vi "CM_Packet_To_Processed_Bytes.vi"(3 "error in (no error)":errorcluster, 4 "CM Params":T5, 5 "CM Packet In":T1) -> (0 "error out":errorcluster, 1 "Processed Bytes":u8[](array[numeric]), 2 "CM Packet Out":T1)   [LabVIEW 2017]
uses:
  Controls/Packet/Packet.ctl
  Controls/Packet/Packet_Direction.ctl
  Controls/Packet/Packet_Type.ctl
  Controls/Packet/Packet_Priority.ctl
  Controls/Control Packets/CM_Param.ctl
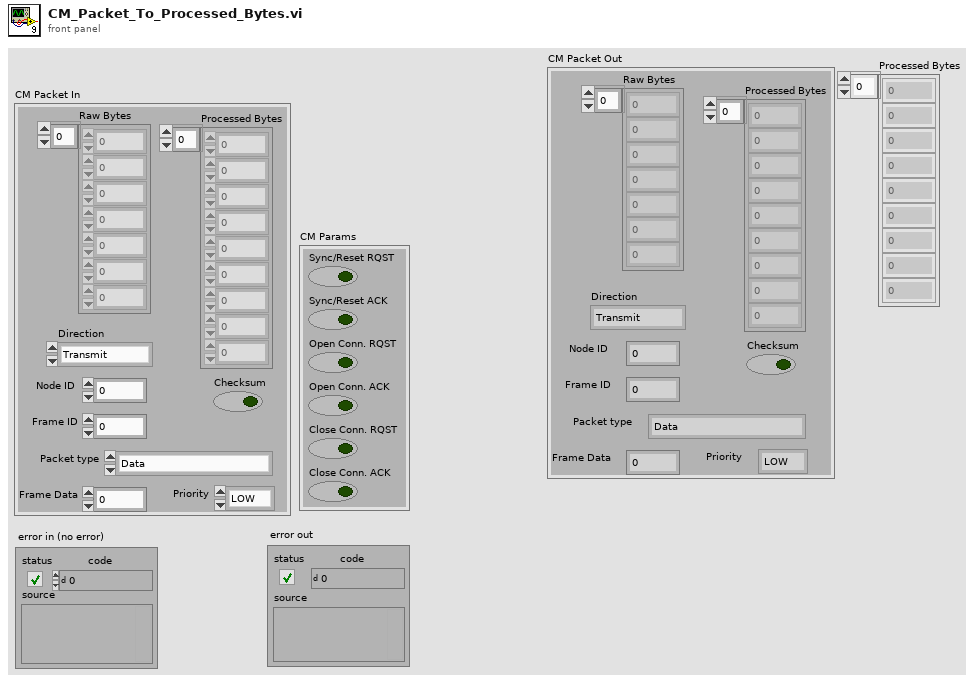
[diagram p1: front panel]
types:
  T1 = typedef "Packet.ctl" = cluster{"Raw Bytes":u8[], "Checksum":bool, "Direction":T2, "Processed Bytes":u8[], "Node ID":u8, "Packet type":T3, "Frame Data":u32, "Priority":T4, "Frame ID":u8}
  T2 = typedef "Packet_Direction.ctl" = enum16{"Transmit", "Receive", "Bidirectional"}
  T3 = typedef "Packet_Type.ctl" = enum16{"Data", "Connection Management", "Remote Request", "Error/Status"}
  T4 = typedef "Packet_Priority.ctl" = enum16{"LOW", "HIGH"}
  T5 = typedef "CM_Param.ctl" = cluster{"Sync/Reset RQST":bool, "Sync/Reset ACK":bool, "Open Conn. RQST":bool, "Open Conn. ACK":bool, "Close Conn. RQST":bool, "Close Conn. ACK":bool}
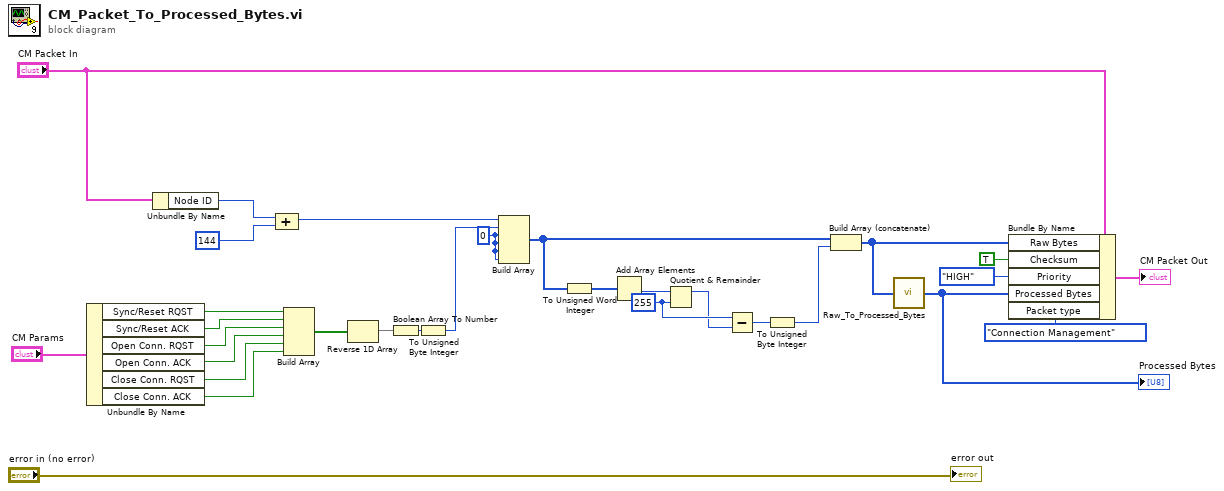
[diagram p0: block diagram]
diagram:
  w13 = u16 255 ("y")
  w17 = u8 0 ("element")
  n1 = Unbundle By Name("CM Params") -> ("Sync/Reset RQST"=w27:bool, "Sync/Reset ACK"=w26:bool, "Open Conn. RQST"=w25:bool, "Open Conn. ACK"=w24:bool, "Close Conn. RQST"=w23:bool, "Close Conn. ACK"=w22:bool)
  n2 = Unbundle By Name("CM Packet In") -> ("Node ID"=w30:u8)
  n3 = Compound Arithmetic op=ADD(w30, u8 144 ("value")) -> (w20:u8)
  n4 = Build Array(w27, w26, w25, w24, w23, w22) -> (w21:bool[])
  n5 = Reverse 1D Array(array=w21) -> (reversed array=w19:bool[])
  n6 = Boolean Array To Number(Boolean array=w19) -> (number=w18:u32)
  n7 = To Unsigned Byte Integer(number=w18) -> (unsigned 8bit integer=w16:u8)
  n8 = Build Array(w20, w16, w17, w17, w17, w17) -> (w11:u8[])
  n9 = To Unsigned Word Integer(number=w11) -> (unsigned 16bit integer=w15:u16[])
  n10 = Add Array Elements(numeric array=w15) -> (sum=w14:u16)
  n11 = Quotient & Remainder(x=w14, y=w13) -> (x-y*floor(x/y)=w12:u16)  [unwired: 1 out]
  n12 = Subtract(x=w13, y=w12) -> (x-y=w10:u16)
  n13 = To Unsigned Byte Integer(number=w10) -> (unsigned 8bit integer=w9:u8)
  n14 = Build Array (concatenate)(w11, w9) -> (w6:u8[])
  n15 = call "Raw_To_Processed_Bytes.vi"("Raw Bytes"=w6) -> ("Processed Bytes"=w3:u8[])
  "Processed Bytes" <- w3
  n16 = Bundle By Name(cluster="CM Packet In", "Raw Bytes"=w6, "Checksum"=TRUE, "Priority"=Packet_Priority."HIGH", "Processed Bytes"=w3, "Packet type"=Packet_Type."Connection Management") -> (→"CM Packet Out":T1)
  "error out" <- "error in (no error)"
